vi "ClientLabView_V2.vi"(5 "?":bool, 6 "Quadre d'instruments":T2={"Missatge a enviar"="No enviar res", "Enviar"=FALSE, "Temps de mostratge"=1.0, "Nombre de mostres mitjana"=1.0, "Adreça IP"=""} {"Nombre de mostres mitjana" min=1.0 max=9.0; "Temps de mostratge" min=1.0 max=20.0}, 7 "?":bool) -> (0 "Historial de mostres":dbl(graph), 1 "Mostra més antiga":dbl, 2 "Temperatura Mínima":string, 3 "Temperatura Màxima":string, 4 "Nombre de mostres":string)   [LabVIEW 2019]
uses:
  Control 1.ctl
panel:
  # "Control Simulació"
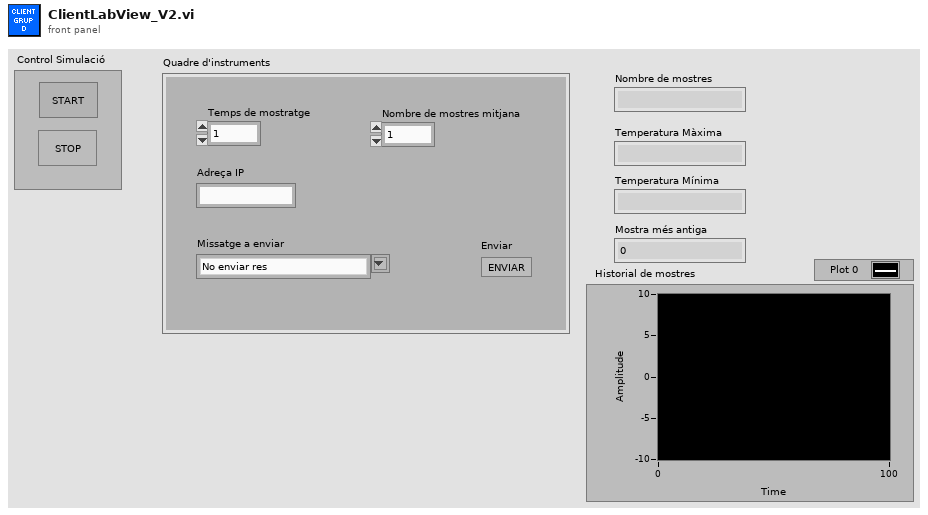
[diagram p1: front panel]
types:
  T1 = typedef "Control 1.ctl" = string
  T2 = cluster{"Missatge a enviar":T1, "Enviar":bool, "Temps de mostratge":dbl, "Nombre de mostres mitjana":dbl, "Adreça IP":string}
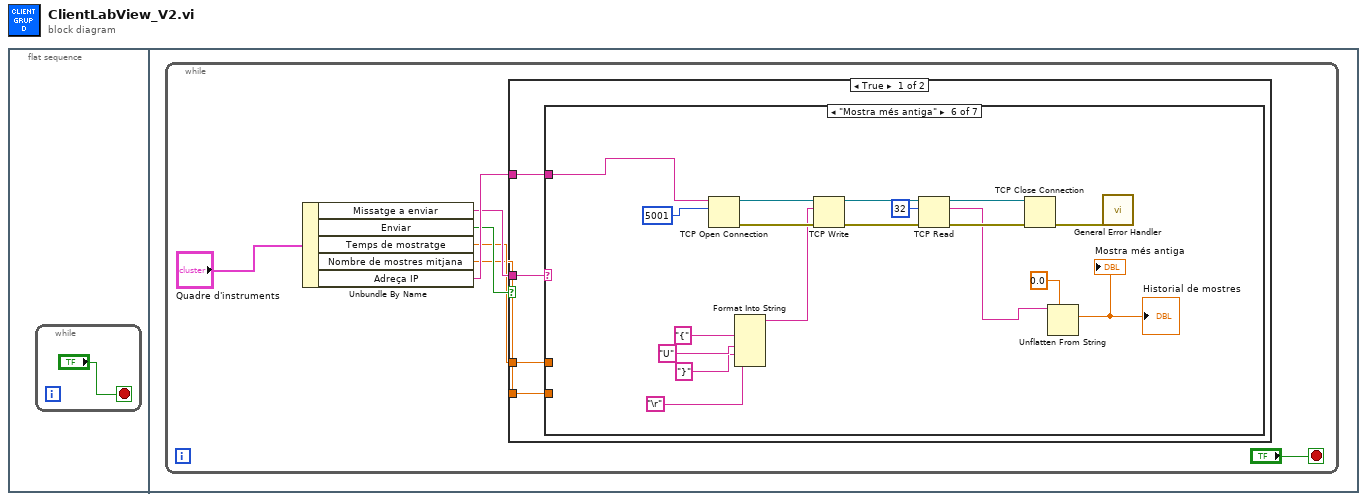
[diagram p0: block diagram]
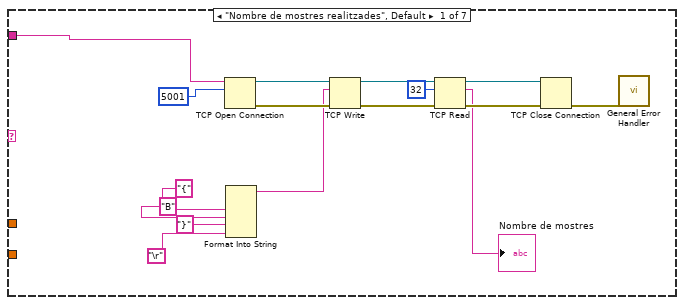
[diagram p2: hidden frame]
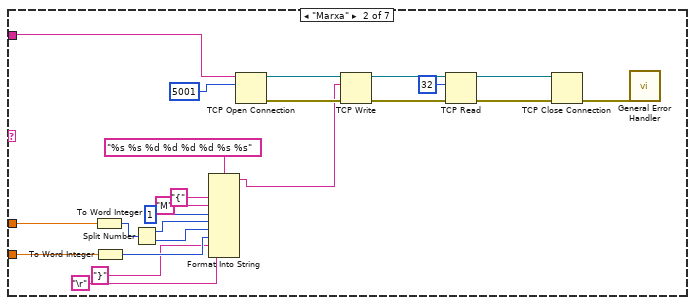
[diagram p3: hidden frame]
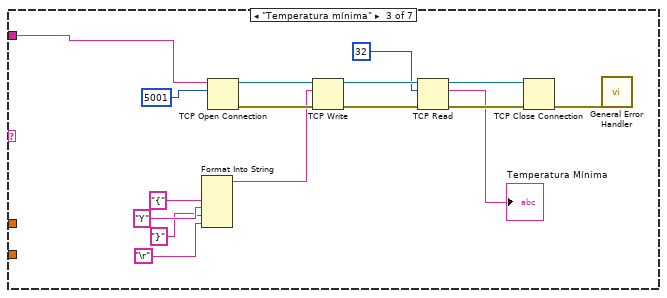
[diagram p4: hidden frame]
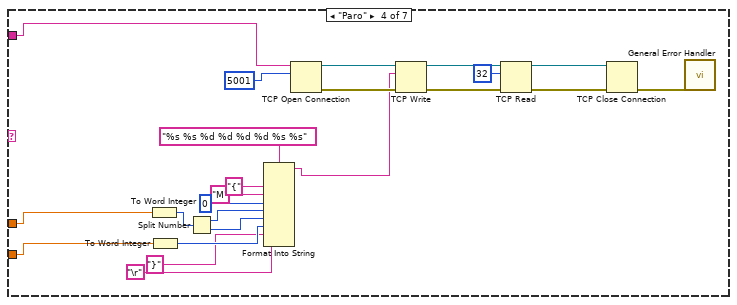
[diagram p5: hidden frame]
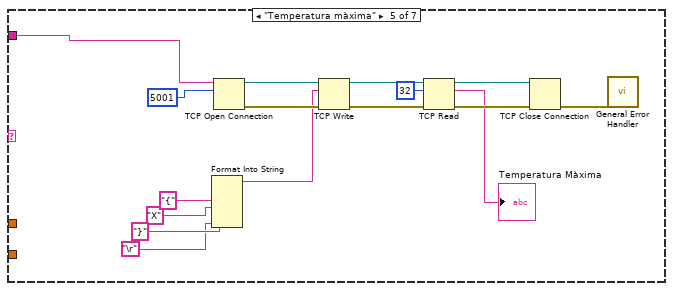
[diagram p6: hidden frame]
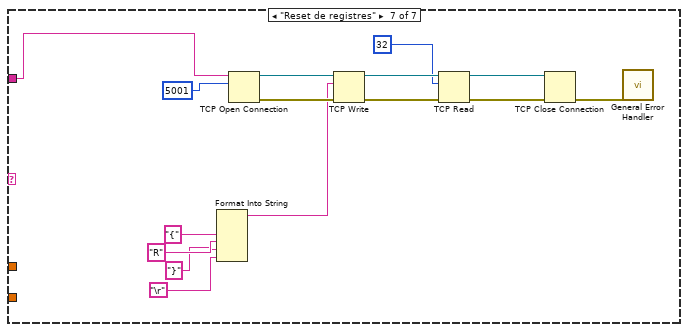
[diagram p7: hidden frame]
diagram:
  n1 = flat-sequence {
    frame #0 {
      n2 = while {
        stop <- "?" stop-if-true
      }
    }
    frame #1 {
      n3 = while {
        stop <- "?" stop-if-true
        n4 = Unbundle By Name("Quadre d'instruments") -> ("Missatge a enviar"=w6:T1, "Enviar"=w5:bool, "Temps de mostratge"=w4:dbl, "Nombre de mostres mitjana"=w3:dbl, "Adreça IP"=w7:string)
        n5 = case shown="True" w5 {
          tunnel: w7 -> [w12 _]
          tunnel: w6 -> [w11 _]
          tunnel: w4 -> [w10 _]
          tunnel: w3 -> [w9 _]
          frame True {
            n6 = case shown="\"Mostra més antiga\"" w11 {
              tunnel: w12 -> [w15 w42 w54 w70 w93 w111 w125]
              tunnel: w10 -> [_ w30 _ w69 _ _ _]
              tunnel: w9 -> [_ w29 _ w68 _ _ _]
              frame "Nombre de mostres realitzades", Default {
                n7 = TCP Open Connection(address=w15, remote port or service name=u16 5001) -> (connection ID=w19:refnum<k5>, error out=w18:errorcluster)  [unwired: 3 in]
                n8 = Format Into String("{", "B", "}", "\r") -> (resulting string=w16:string)  [unwired: 3 in, 1 out]
                n9 = TCP Write(connection ID=w19, data in=w16, error in (no error)=w18) -> (connection ID out=w20:refnum<k5>, error out=w22:errorcluster)  [unwired: 1 in, 1 out]
                n10 = TCP Read(connection ID=w20, bytes to read=32, error in (no error)=w22) -> (connection ID out=w21:refnum<k5>, data out=→"Nombre de mostres":string, error out=w23:errorcluster)  [unwired: 2 in]
                n11 = TCP Close Connection(connection ID=w21, error in (no error)=w23) -> (error out=w24:errorcluster)  [unwired: 1 in, 1 out]
                n12 = call <vilib>:"General Error Handler.vi"("error in (no error)"=w24) -> ()  [unwired: 10 in, 5 out]
              }
              frame "Marxa" {
                n13 = To Word Integer(number=w30) -> (16bit integer=w37:i16)
                n14 = To Word Integer(number=w29) -> (16bit integer=w34:i16)
                n15 = Split Number(x=w37) -> (hi(x)=w36:u8, lo(x)=w35:u8)
                n16 = Format Into String(format string="%s %s %d %d %d %d %s %s", "{", "M" ("input 2"), 1 ("input 3"), w36, w35, w34, "}", "\r") -> (resulting string=w31:string)  [unwired: 2 in, 1 out]
                n17 = TCP Open Connection(address=w42, remote port or service name=u16 5001) -> (connection ID=w46:refnum<k5>, error out=w45:errorcluster)  [unwired: 3 in]
                n18 = TCP Write(connection ID=w46, data in=w31, error in (no error)=w45) -> (connection ID out=w47:refnum<k5>, error out=w49:errorcluster)  [unwired: 1 in, 1 out]
                n19 = TCP Read(connection ID=w47, bytes to read=32, error in (no error)=w49) -> (connection ID out=w48:refnum<k5>, error out=w50:errorcluster)  [unwired: 2 in, 1 out]
                n20 = TCP Close Connection(connection ID=w48, error in (no error)=w50) -> (error out=w51:errorcluster)  [unwired: 1 in, 1 out]
                n21 = call <vilib>:"General Error Handler.vi"("error in (no error)"=w51) -> ()  [unwired: 10 in, 5 out]
              }
              frame "Temperatura mínima" {
                n22 = Format Into String("{", "Y", "}", "\r") -> (resulting string=w55:string)  [unwired: 3 in, 1 out]
                n23 = TCP Open Connection(address=w54, remote port or service name=u16 5001) -> (connection ID=w58:refnum<k5>, error out=w57:errorcluster)  [unwired: 3 in]
                n24 = TCP Write(connection ID=w58, data in=w55, error in (no error)=w57) -> (connection ID out=w59:refnum<k5>, error out=w61:errorcluster)  [unwired: 1 in, 1 out]
                n25 = TCP Read(connection ID=w59, bytes to read=32, error in (no error)=w61) -> (connection ID out=w60:refnum<k5>, data out=→"Temperatura Mínima":string, error out=w62:errorcluster)  [unwired: 2 in]
                n26 = TCP Close Connection(connection ID=w60, error in (no error)=w62) -> (error out=w63:errorcluster)  [unwired: 1 in, 1 out]
                n27 = call <vilib>:"General Error Handler.vi"("error in (no error)"=w63) -> ()  [unwired: 10 in, 5 out]
              }
              frame "Paro" {
                n28 = To Word Integer(number=w69) -> (16bit integer=w77:i16)
                n29 = To Word Integer(number=w68) -> (16bit integer=w74:i16)
                n30 = Split Number(x=w77) -> (hi(x)=w76:u8, lo(x)=w75:u8)
                n31 = Format Into String(format string="%s %s %d %d %d %d %s %s", "{", "M" ("input 2"), 0 ("input 3"), w76, w75, w74, "}", "\r") -> (resulting string=w71:string)  [unwired: 2 in, 1 out]
                n32 = TCP Open Connection(address=w70, remote port or service name=u16 5001) -> (connection ID=w85:refnum<k5>, error out=w84:errorcluster)  [unwired: 3 in]
                n33 = TCP Write(connection ID=w85, data in=w71, error in (no error)=w84) -> (connection ID out=w86:refnum<k5>, error out=w88:errorcluster)  [unwired: 1 in, 1 out]
                n34 = TCP Read(connection ID=w86, bytes to read=32, error in (no error)=w88) -> (connection ID out=w87:refnum<k5>, error out=w89:errorcluster)  [unwired: 2 in, 1 out]
                n35 = TCP Close Connection(connection ID=w87, error in (no error)=w89) -> (error out=w90:errorcluster)  [unwired: 1 in, 1 out]
                n36 = call <vilib>:"General Error Handler.vi"("error in (no error)"=w90) -> ()  [unwired: 10 in, 5 out]
              }
              frame "Temperatura màxima" {
                n37 = Format Into String("{", "X", "}", "\r") -> (resulting string=w94:string)  [unwired: 3 in, 1 out]
                n38 = TCP Open Connection(address=w93, remote port or service name=u16 5001) -> (connection ID=w97:refnum<k5>, error out=w96:errorcluster)  [unwired: 3 in]
                n39 = TCP Write(connection ID=w97, data in=w94, error in (no error)=w96) -> (connection ID out=w98:refnum<k5>, error out=w100:errorcluster)  [unwired: 1 in, 1 out]
                n40 = TCP Read(connection ID=w98, bytes to read=32, error in (no error)=w100) -> (connection ID out=w99:refnum<k5>, data out=→"Temperatura Màxima":string, error out=w101:errorcluster)  [unwired: 2 in]
                n41 = TCP Close Connection(connection ID=w99, error in (no error)=w101) -> (error out=w102:errorcluster)  [unwired: 1 in, 1 out]
                n42 = call <vilib>:"General Error Handler.vi"("error in (no error)"=w102) -> ()  [unwired: 10 in, 5 out]
              }
              frame "Mostra més antiga" {
                n43 = TCP Open Connection(address=w111, remote port or service name=u16 5001) -> (connection ID=w119:refnum<k5>, error out=w120:errorcluster)  [unwired: 3 in]
                n44 = Format Into String("{", "U", "}", "\r") -> (resulting string=w112:string)  [unwired: 3 in, 1 out]
                n45 = TCP Write(connection ID=w119, data in=w112, error in (no error)=w120) -> (connection ID out=w118:refnum<k5>, error out=w116:errorcluster)  [unwired: 1 in, 1 out]
                n46 = TCP Read(connection ID=w118, bytes to read=32, error in (no error)=w116) -> (connection ID out=w117:refnum<k5>, data out=w109:string, error out=w115:errorcluster)  [unwired: 2 in]
                n47 = TCP Close Connection(connection ID=w117, error in (no error)=w115) -> (error out=w114:errorcluster)  [unwired: 1 in, 1 out]
                n48 = Unflatten From String(type=0.0, binary string=w109) -> (value=→"Historial de mostres" →"Mostra més antiga":dbl)  [unwired: 3 in, 2 out]
                n49 = call <vilib>:"General Error Handler.vi"("error in (no error)"=w114) -> ()  [unwired: 10 in, 5 out]
              }
              frame "Reset de registres" {
                n50 = Format Into String("{", "R", "}", "\r") -> (resulting string=w126:string)  [unwired: 3 in, 1 out]
                n51 = TCP Open Connection(address=w125, remote port or service name=u16 5001) -> (connection ID=w130:refnum<k5>, error out=w129:errorcluster)  [unwired: 3 in]
                n52 = TCP Write(connection ID=w130, data in=w126, error in (no error)=w129) -> (connection ID out=w131:refnum<k5>, error out=w133:errorcluster)  [unwired: 1 in, 1 out]
                n53 = TCP Read(connection ID=w131, bytes to read=32, error in (no error)=w133) -> (connection ID out=w132:refnum<k5>, error out=w134:errorcluster)  [unwired: 2 in, 1 out]
                n54 = TCP Close Connection(connection ID=w132, error in (no error)=w134) -> (error out=w135:errorcluster)  [unwired: 1 in, 1 out]
                n55 = call <vilib>:"General Error Handler.vi"("error in (no error)"=w135) -> ()  [unwired: 10 in, 5 out]
              }
            }
          }
          frame False {
          }
        }
      }
    }
  }
